vi "resample_centerline.vi"(0 "Last Centerline (last centroid)":sgl[][](array[numeric]), 1 "Centroid (bounding rectangle)":dbl[][](array[numeric]), 2 "Centerline Pixels":i32[][](array[numeric]), 3 "Sample Points":i32, 4 "current centroid (camera origin)":sgl[](array[numeric])) -> (5 "Centerline (camera origin)":sgl[][](array[numeric]), 6 "Centerline (bounding rectangle)":sgl[][](array[numeric]), 7 "Centerline found?":bool)   [LabVIEW 2019]
uses:
  <vilib>/gmath/interp.llb/Search Ordered Table.vi
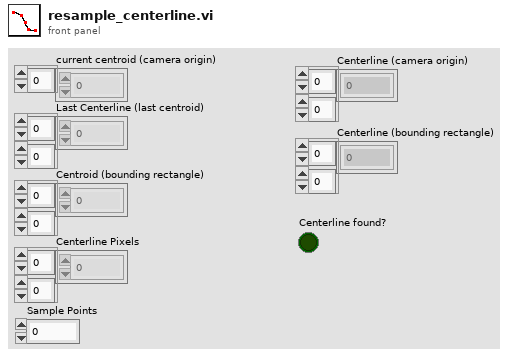
[diagram p1: front panel]
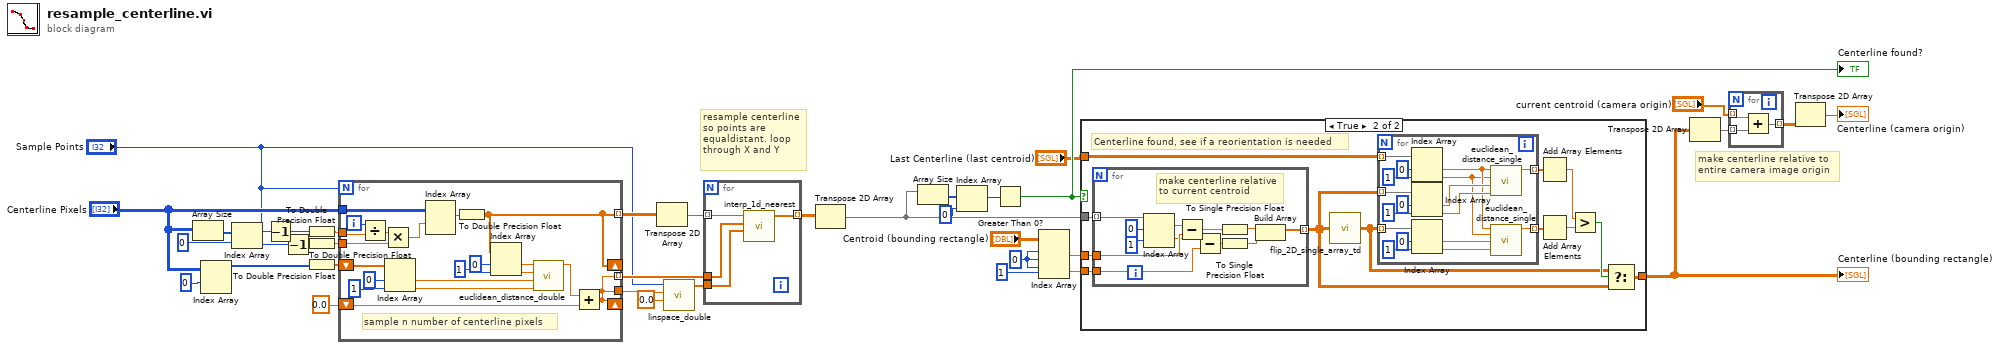
[diagram p0: block diagram]
diagram:
  w12 = 0 ("index (row)")
  # "make centerline relative to\nentire camera image origin"
  # "resample centerline\nso points are\nequaldistant. loop\nthrough X and Y"
  n1 = Array Size(array="Centerline Pixels") -> (size(s)=w34:i32[])
  n2 = Index Array(array="Centerline Pixels", index (row)=0) -> (element=w28:i32[])  [unwired: 1 in]
  n3 = Index Array(array=w34, index=0) -> (element=w23:i32)
  n4 = Decrement(x="Sample Points") -> (x-1=w22:i32)
  n5 = Decrement(x=w23) -> (x-1=w20:i32)
  n6 = To Double Precision Float(number=w22) -> (double precision float=w21:dbl)
  n7 = To Double Precision Float(number=w20) -> (double precision float=w19:dbl)
  n8 = To Double Precision Float(number=w28) -> (double precision float=w27:dbl[])
  n9 = for {
    N: "Sample Points" -> [_]
    tunnel: "Centerline Pixels" -> [w54]
    tunnel: [w43] -> w30 mode=indexing
    shift-right: [w43] -> _
    shift-left: w27 -> [w49]
    shift-right: [w40] -> _
    shift-left: 0.0 ("Distance") -> [w41]
    tunnel: [w40] -> w25 mode=indexing
    tunnel: [w40] -> w24
    tunnel: w21 -> [w39]
    tunnel: w19 -> [w37]
    i -> [w56]
    # "sample n number of centerline pixels"
    n10 = Divide(x=w56, y=w39) -> (x/y=w55:dbl)
    n11 = Multiply(x=w55, y=w37) -> (x*y=w38:dbl)
    n12 = Index Array(array=w49, index #1=0 ("index"), index #2=1 ("index")) -> (element #1=w45:dbl, element #2=w44:dbl)
    n13 = Index Array(array=w54, index (row)=w38) -> (element=w48:i32[])  [unwired: 1 in]
    n14 = To Double Precision Float(number=w48) -> (double precision float=w43:dbl[])
    n15 = Index Array(array=w43, index #1=0 ("index"), index #2=1 ("index")) -> (element #1=w47:dbl, element #2=w46:dbl)
    n16 = call "euclidean_distance_double.vi"("Point 2 Y"=w44, "Point 2 X"=w45, "Point 1 Y"=w46, "Point 1 X"=w47) -> ("Distance"=w42:dbl)  [unwired: 7 in]
    n17 = Add(x=w42, y=w41) -> (x+y=w40:dbl)
  }
  n18 = Transpose 2D Array(2D array=w30) -> (transposed array=w36:dbl[][])
  n19 = call "linspace_double.vi"("start"=0.0, "end"=w24, "samples"="Sample Points") -> ("Ramp Pattern"=w31:dbl[])  [unwired: 8 in]
  n20 = for {
    tunnel: w36 -> [w57] mode=indexing
    tunnel: w25 -> [w60]
    tunnel: [w59] -> w35 mode=indexing
    tunnel: w31 -> [w58]
    n21 = call "interp_1d_nearest.vi"("xi"=w58, "X"=w60, "Y"=w57) -> ("yi"=w59:dbl[])  [unwired: 8 in]
  }
  n22 = Transpose 2D Array(2D array=w35) -> (transposed array=w5:dbl[][])
  n23 = Array Size(array=w5) -> (size(s)=w16:i32[])
  n24 = Index Array(array=w16, index=0) -> (element=w13:i32)
  n25 = Greater Than 0?(x=w13) -> (x > 0?=w8:bool)
  "Centerline found?" <- w8
  n26 = Index Array(array="Centroid (bounding rectangle)", index (row) #1=w12, index (col) #1=w12, index (row) #2=w12, index (col) #2=1 ("disabled index (col)")) -> (element #1=w7:dbl, element #2=w6:dbl)
  n27 = case shown="True" w8 {
    tunnel: "Last Centerline (last centroid)" -> [w61 w73]
    tunnel: [w61 w67] -> w9
    tunnel: w5 -> [_ w66]
    tunnel: w7 -> [_ w65]
    tunnel: w6 -> [_ w64]
    frame False {
      # "Centerline not found, use last"
    }
    frame True {
      # "Centerline found, see if a reorientation is needed"
      n28 = for {
        tunnel: w66 -> [w85] mode=indexing
        tunnel: w65 -> [w82]
        tunnel: w64 -> [w81]
        tunnel: [w76] -> w62 mode=indexing
        # "make centerline relative\nto current centroid"
        n29 = Index Array(array=w85, index #1=0, index #2=1) -> (element #1=w80:dbl, element #2=w79:dbl)
        n30 = Subtract(x=w80, y=w82) -> (x-y=w78:dbl)
        n31 = Subtract(x=w79, y=w81) -> (x-y=w77:dbl)
        n32 = To Single Precision Float(number=w78) -> (single precision float=w75:sgl)
        n33 = To Single Precision Float(number=w77) -> (single precision float=w74:sgl)
        n34 = Build Array(w75, w74) -> (w76:sgl[])
      }
      n35 = call "flip_2D_single_array_td.vi"("Centerline"=w62) -> ("Array Flipped Top Down"=w63:sgl[][])
      n36 = for {
        tunnel: w73 -> [w98] mode=indexing
        tunnel: [w97] -> w72 mode=indexing
        tunnel: w63 -> [w91] mode=indexing
        tunnel: w62 -> [w94] mode=indexing
        tunnel: [w86] -> w71 mode=indexing
        n37 = Index Array(array=w98, index #1=0 ("index"), index #2=1 ("index")) -> (element #1=w90:sgl, element #2=w89:sgl)
        n38 = Index Array(array=w94, index #1=0 ("index"), index #2=1 ("index")) -> (element #1=w96:sgl, element #2=w95:sgl)
        n39 = Index Array(array=w91, index #1=0 ("index"), index #2=1 ("index")) -> (element #1=w88:sgl, element #2=w87:sgl)
        n40 = call "euclidean_distance_single.vi"("Point 2 Y"=w95, "Point 2 X"=w96, "Point 1 Y"=w89, "Point 1 X"=w90) -> ("Distance"=w97:sgl)  [unwired: 7 in]
        n41 = call "euclidean_distance_single.vi"("Point 2 Y"=w87, "Point 2 X"=w88, "Point 1 Y"=w89, "Point 1 X"=w90) -> ("Distance"=w86:sgl)  [unwired: 7 in]
      }
      n42 = Add Array Elements(numeric array=w72) -> (sum=w70:sgl)
      n43 = Add Array Elements(numeric array=w71) -> (sum=w69:sgl)
      n44 = Greater?(x=w70, y=w69) -> (0:w68:bool)
      n45 = Select(t=w63, s=w68, f=w62) -> (s? t:f=w67:sgl[][])
    }
  }
  "Centerline (bounding rectangle)" <- w9
  n46 = Transpose 2D Array(2D array=w9) -> (transposed array=w11:sgl[][])
  n47 = for {
    tunnel: w11 -> [w104] mode=indexing
    tunnel: "current centroid (camera origin)" -> [w105] mode=indexing
    tunnel: [w103] -> w10 mode=indexing
    n48 = Add(x=w105, y=w104) -> (x+y=w103:sgl[])
  }
  n49 = Transpose 2D Array(2D array=w10) -> (transposed array=→"Centerline (camera origin)":sgl[][])
